vi "Module Type.vi"(11 "DAQmxDI in":refnum<class " DAQmxDI Port.lvclass">) -> (2 "Module Type":string)   [LabVIEW 2020, in " DAQmxDI Port.lvclass"]
uses:
   DAQmxDI Port.lvclass
   DAQmxDI Port.lvclass/ DAQmxDI Port.ctl
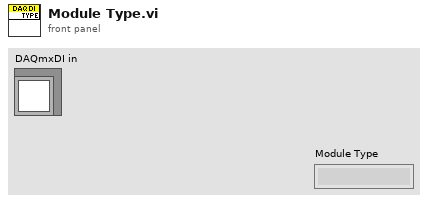
[diagram p1: front panel]
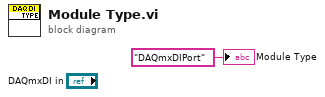
[diagram p0: block diagram]
diagram:
  "Module Type" <- "DAQmxDIPort" ("Module Type")
